vi "Hyperbolamodel.vi"(3 "输出控制":T1, 4 "数据":variant, 5 "Z":dbl[](array[numeric]), 6 "a":dbl[](array[numeric])) -> (0 "error out":cluster{"状态":bool, "代码":i32, "源":string} caption="错误输出", 1 "f'(X,a)":dbl[][](array[numeric]), 2 "f(X,a)":dbl[](array[numeric]))   [LabVIEW 2018]
doc: "高斯光束双曲线模型"
uses:
  <vilib>/gmath/NumericalOptimization/LM_output select.ctl
  <vilib>/gmath/NI_Gmath.lvlib
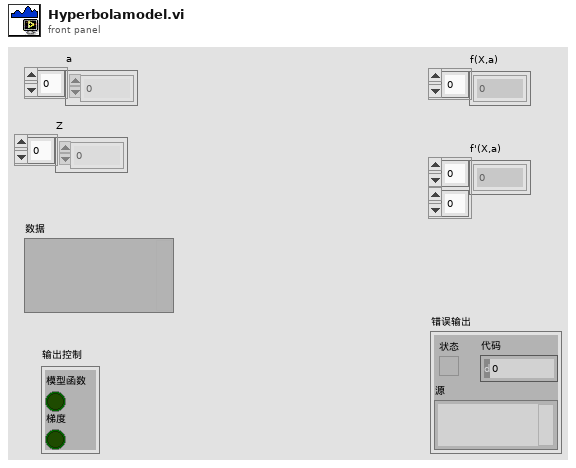
[diagram p1: front panel]
types:
  T1 = typedef "NI_Gmath.lvlib/LM_output select.ctl" = cluster{"model function":bool, "gradient":bool}
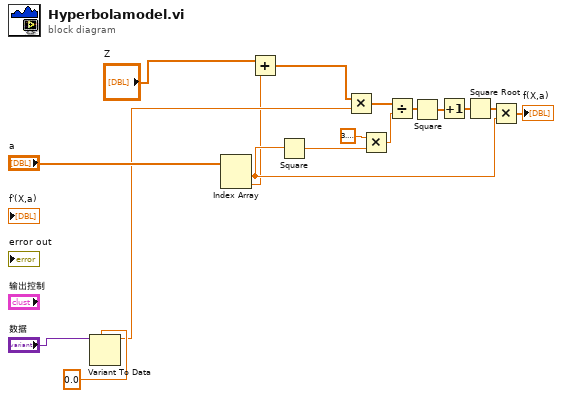
[diagram p0: block diagram]
diagram:
  n1 = Variant To Data(type=0.0, Variant="数据") -> (data=w5:dbl)  [unwired: 1 in, 1 out]
  n2 = Index Array(array="a") -> (element #1=w14:dbl, element #2=w2:dbl)  [unwired: 2 in]
  n3 = Add(x="Z", y=w2) -> (x+y=w1:dbl[])
  n4 = Square(x=w14) -> (x^2=w13:dbl)
  n5 = Multiply(x=w1, y=w5) -> (x*y=w16:dbl[])
  n6 = Multiply(x=3.141592653589793, y=w13) -> (x*y=w12:dbl)
  n7 = Divide(x=w16, y=w12) -> (x/y=w11:dbl[])
  n8 = Square(x=w11) -> (x^2=w10:dbl[])
  n9 = Increment(x=w10) -> (x+1=w9:dbl[])
  n10 = Square Root(x=w9) -> (sqrt(x)=w8:dbl[])
  n11 = Multiply(x=w8, y=w14) -> (x*y=→"f(X,a)":dbl[])
